vi "ProcessSensorData.vi"(8 "error in (no error)":errorcluster, 10 "clSensorData":T1, 11 "Class In":refnum<class "FFT.lvclass">) -> (0 "error out":errorcluster, 3 "Class Out":refnum<class "FFT.lvclass">)   [LabVIEW 2014, in "AnalysisPlugins.lvlib" / "FFT.lvclass"]
uses:
  FFT.lvclass
  AnalysisPluginBaseClass/Typedefs/clSensorData.ctl
  AnalysisPluginBaseClass/AnalysisPluginsBase.lvclass/AnalysisPluginsBase.ctl
  AnalysisPluginBaseClass/Accessors/Read AnalysisTime.vi
  AnalysisPluginBaseClass/Accessors/Write AnalysisTime.vi
  AnalysisPluginBaseClass/AnalysisPluginsBase.lvclass
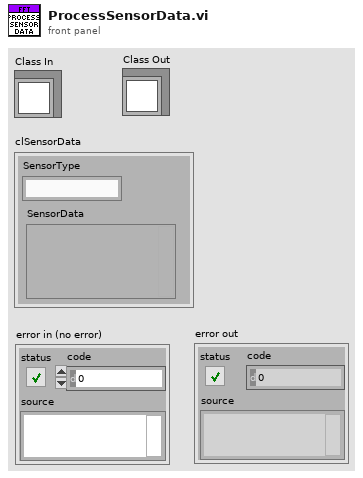
[diagram p1: front panel]
types:
  T1 = typedef "AnalysisPlugins.lvlib/AnalysisPluginsBase.lvclass/clSensorData.ctl" = cluster{"SensorType":string, "SensorData":variant}
  T2 = typedef "AnalysisPlugins.lvlib/PmuAnalysis.lvclass/clAnalysisConfig.ctl" = cluster{"F0":u32, "SettlingTime":dbl, "AnalysisCycles":dbl, "SampleRate":dbl, "NumChannels":u32, "TsOffset":enum16{"start", "middle", "end"}}
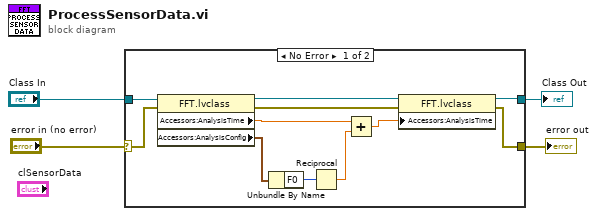
[diagram p0: block diagram]
diagram:
  n1 = case shown="No Error" "error in (no error)" {
    selector: "error in (no error)" -> [w14 w16]
    tunnel: "Class In" -> [w15 w17]
    tunnel: [w6 w17] -> w2
    tunnel: [w5 w16] -> w1
    frame No Error {
      n2 = property class="FFT.lvclass"(reference=w15, error in=w14) -> (reference out=w9:refnum<class "FFT.lvclass">, error out=w8:errorcluster, "Accessors:AnalysisTime"=w11:dbl, "Accessors:AnalysisConfig"=w13:T2)
      n3 = Unbundle By Name(w13) -> ("F0"=w12:u32)
      n4 = Reciprocal(x=w12) -> (1/x=w10:dbl)
      n5 = Add(x=w11, y=w10) -> (x+y=w7:dbl)
      n6 = property class="FFT.lvclass"(reference=w9, error in=w8, "Accessors:AnalysisTime"=w7) -> (reference out=w6:refnum<class "FFT.lvclass">, error out=w5:errorcluster)
    }
    frame Error {
    }
  }
  "Class Out" <- w2
  "error out" <- w1
